vi "Orb_Initialize.vi"(2 "traceLevel":i16, 9 "error in (no error)":errorcluster) -> (6 "error out":errorcluster)   [LabVIEW 2009]
uses:
  Orb_Global.vi
  lib/lvrtc.dll
panel:
  out "return type":i32
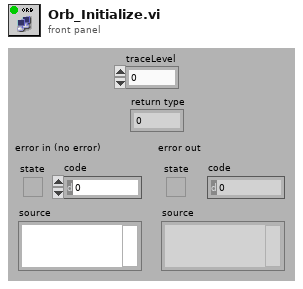
[diagram p1: front panel]
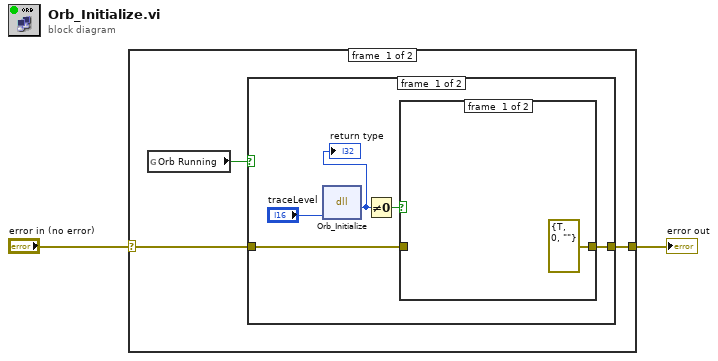
[diagram p0: block diagram]
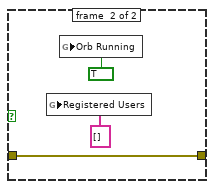
[diagram p2: hidden frame]
diagram:
  n1 = case shown="No Error" "error in (no error)" {
    selector: "error in (no error)" -> [w3 w16]
    tunnel: [w5 w16] -> w2
    frame #0 {
      n2 = global read "Orb_Global.vi" "Orb Running"() -> (w4:bool)
      n3 = case shown="False" w4 {
        tunnel: w3 -> [w8 w15]
        tunnel: [w7 w15] -> w5
        frame #0 {
          n4 = dll-call lib="C:/Ohana/LV2009/OhanaOS-LV81/Instruments/RTC/Api/lib/lvrtc.dll" fn="Orb_Initialize"("debug"="traceLevel") -> ("return type"=w6:i32)  [unwired: 4 in, 2 out]
          "return type" <- w6
          n5 = Not Equal To 0?(x=w6) -> (x != 0?=w9:bool)
          n6 = case shown="False" w9 {
            tunnel: w8 -> [_ w12]
            tunnel: [errorcluster {"status"=TRUE, "code"=0, "source"=""} ("error IO") w12] -> w7
            frame #0 {
            }
            frame #1 {
              n7 = global write "Orb_Global.vi" "Registered Users"(string[] [] ("Registered Users")) -> ()
              n8 = global write "Orb_Global.vi" "Orb Running"(TRUE ("Orb Running")) -> ()
            }
          }
        }
        frame #1 {
        }
      }
    }
    frame #1 {
    }
  }
  "error out" <- w2
